vi "GetExistingObject.vi"(8 "ErrorIn":errorcluster, 10 "ObjectName":string, 11 "Type":refnum<class>) -> (0 "ErrorOut":errorcluster, 3 "ObjectOut":refnum<class>)   [LabVIEW 2021, in "Application.lvclass"]
doc: "Returns the object from the pool with the specified type and label. If you provide an interface the interface implemenation is returned."
uses:
  Application.lvclass
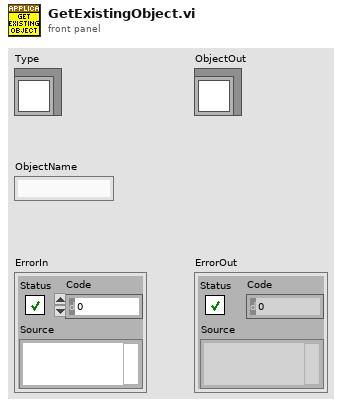
[diagram p1: front panel]
types:
  T1 = typedef "Application.lvclass/ObjectAttributes.ctl" = cluster{"Objects":variant, "BasePath":path, "Application":refnum<class "Application.lvclass">}
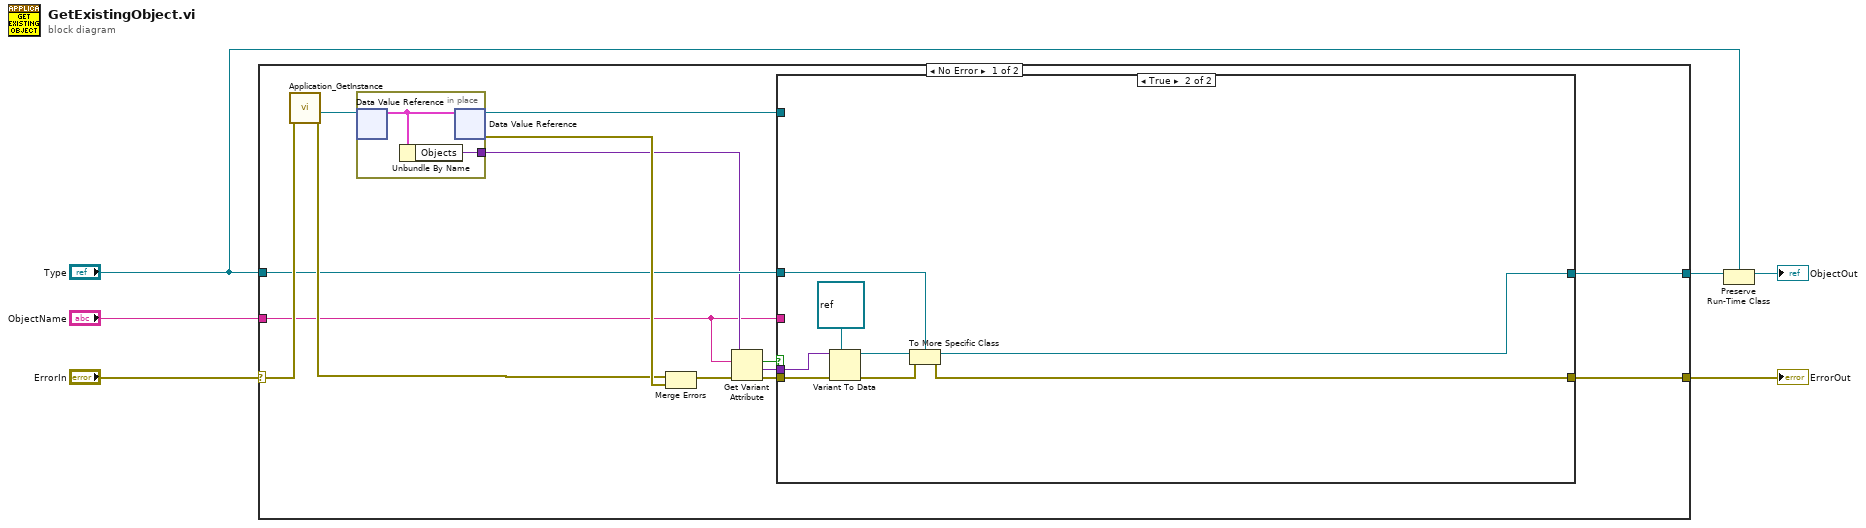
[diagram p0: block diagram]
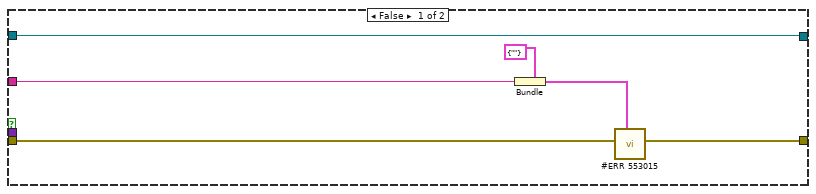
[diagram p2: hidden frame]
diagram:
  n1 = case shown="No Error" "ErrorIn" {
    selector: "ErrorIn" -> [w20 w37]
    tunnel: [w16 w37] -> w5
    tunnel: "ObjectName" -> [w7 _]
    tunnel: "Type" -> [w14 _]
    tunnel: [w13 _] -> w3
    frame No Error {
      n2 = call "Application_GetInstance.vi"("ErrorIn"=w20) -> ("ErrorOut"=w15:errorcluster, "DVRRefOut"=w12:refnum<data-value>)  [unwired: 6 in, 3 out]
      n3 = in-place {
        in-place-border: [w35] -> w9
        n4 = in-place-dvr #1(w12) -> (w36:T1)  [unwired: 1 out]
        n5 = Unbundle By Name(w36) -> ("Objects"=w35:variant)
        n6 = in-place-dvr #1(w36) -> (w8:refnum<data-value>, w19:errorcluster)
      }
      n7 = Merge Errors(w15, w19) -> (w18:errorcluster)
      n8 = Get Variant Attribute(Variant=w9, name=w7, error in=w18) -> (found=w11:bool, value=w10:variant, error out=w17:errorcluster)  [unwired: 1 in, 1 out]
      n9 = case shown="True" w11 {
        tunnel: w17 -> [w26 w34]
        tunnel: w14 -> [w24 w27]
        tunnel: [w25 w32] -> w16
        tunnel: [w24 w28] -> w13
        tunnel: w10 -> [_ w30]
        tunnel: w8 -> [_ _]
        tunnel: w7 -> [w23 _]
        frame False {
          n10 = Bundle(cluster=cluster{"ObjectName":string} {"ObjectName"=""}, "ObjectName"=w23) -> (w22:cluster{"ObjectName":string})
          n11 = call "#ERR 553015"("Data"=w22, "error in (no error)"=w26) -> ("error out"=w25:errorcluster)  [unwired: 9 in]
        }
        frame True {
          n12 = Variant To Data(error in=w34, type=refnum<class> refnum ("Type"), Variant=w30) -> (data=w29:refnum<class>, error out=w33:errorcluster)
          n13 = To More Specific Class(target class=w27, reference=w29, error in=w33) -> (specific class reference=w28:refnum<class>, error out=w32:errorcluster)
        }
      }
    }
    frame Error {
    }
  }
  "ErrorOut" <- w5
  n14 = Preserve Run-Time Class(object in=w3, 2:"Type") -> (object out=→"ObjectOut":refnum<class>)  [unwired: 1 in, 1 out]
